vi "getData.vi"(9 "COM":bool, 10 "VISA name":refnum<visa-resource-name>, 11 "Array":string[](array[string])) -> (2 "return":i32, 3 "Numeric":u16)   [LabVIEW 2016]
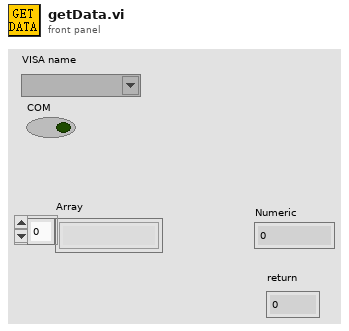
[diagram p1: front panel]
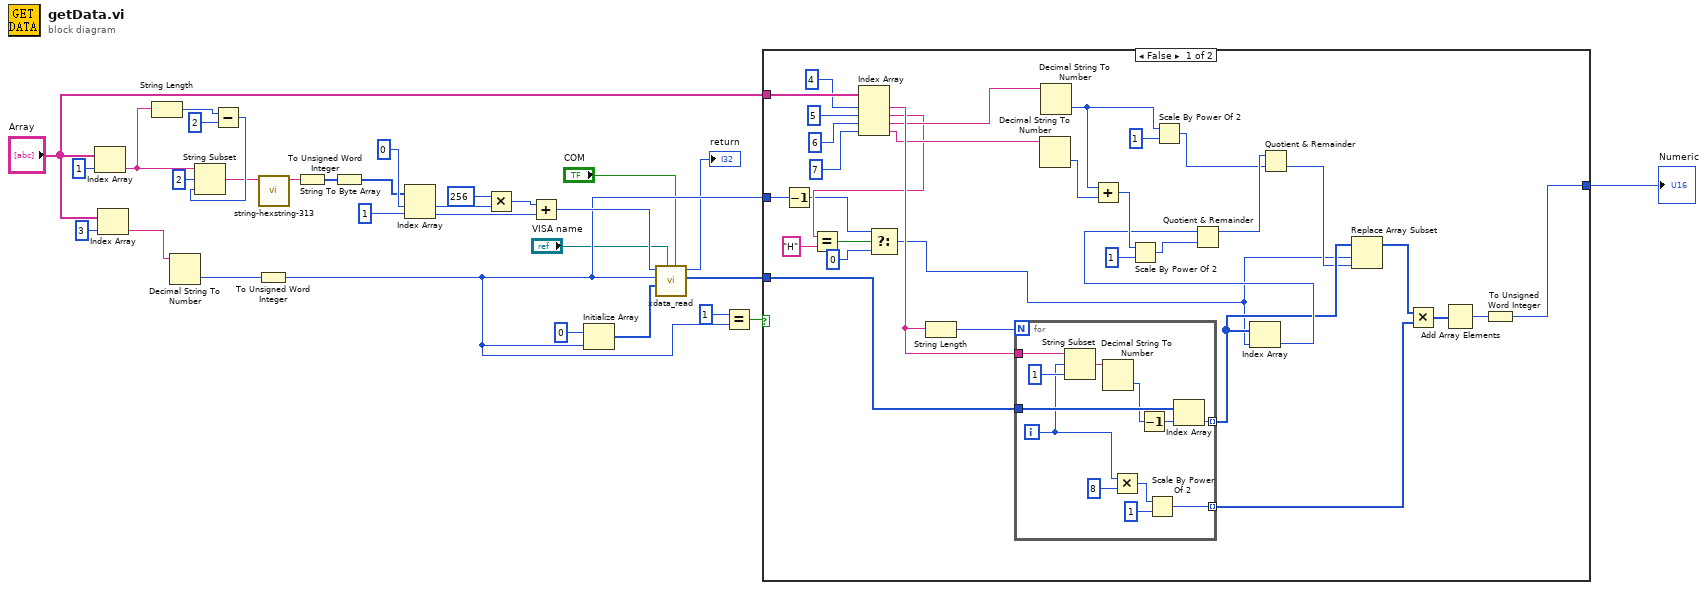
[diagram p0: block diagram]
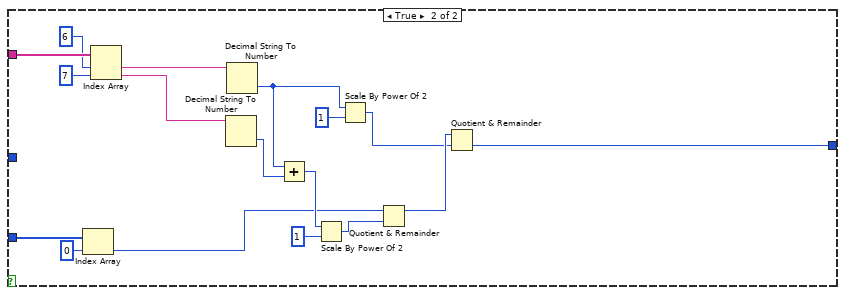
[diagram p2: hidden frame]
diagram:
  n1 = Index Array(array="Array", index=1) -> (element=w30:string)
  n2 = Index Array(array="Array", index=3) -> (element=w14:string)
  n3 = String Length(string=w30) -> (length=w29:i32)
  n4 = Decimal String To Number(string=w14) -> (number=w12:i32)  [unwired: 2 in, 1 out]
  n5 = Subtract(x=w29, y=2) -> (x-y=w27:i32)
  n6 = String Subset(string=w30, offset (0)=2, length (rest)=w27) -> (substring=w25:string)
  n7 = To Unsigned Word Integer(number=w12) -> (unsigned 16bit integer=w4:u16)
  n8 = call "string-hexstring-313.vi"("字符串"=w25) -> ("十六进制整型字符串"=w24:string)  [unwired: 10 in]
  n9 = String To Byte Array(string=w24) -> (unsigned byte array=w23:u8[])
  n10 = To Unsigned Word Integer(number=w23) -> (unsigned 16bit integer=w20:u16[])
  n11 = Index Array(array=w20, index #1=0 ("index"), index #2=1 ("index")) -> (element #1=w19:u16, element #2=w16:u16)
  n12 = Multiply(x=u16 256, y=w19) -> (x*y=w17:u16)
  n13 = Add(x=w17, y=w16) -> (x+y=w13:u16)
  n14 = Initialize Array(u8 0 ("element"), w4) -> (w10:u8[])
  n15 = call "xdata_read.vi"("COM"="COM", "VISA name"="VISA name", "data"=w10, "wLen"=w4, "wAddr"=w13) -> ("data out"=w7:u8[], "return"=→"return":i32)  [unwired: 5 in]
  n16 = Equal?(x=u16 1, y=w4) -> (x = y?=w9:bool)
  n17 = case shown="False" w9 {
    tunnel: w7 -> [w47 w93]
    tunnel: "Array" -> [w64 w91]
    tunnel: [w39 w77] -> w5
    tunnel: w4 -> [w35 _]
    frame False {
      n18 = Decrement(x=w35) -> (x-1=w32:u16)
      n19 = Index Array(array=w64, index #1=4 ("index"), index #2=5 ("index"), index #3=6 ("index"), index #4=7 ("index")) -> (element #1=w50:string, element #2=w38:string, element #3=w49:string, element #4=w48:string)
      n20 = Equal?(x=w38, y="H") -> (x = y?=w36:bool)
      n21 = Select(t=w32, s=w36, f=u16 0) -> (s? t:f=w33:u16)
      n22 = String Length(string=w50) -> (length=w51:i32)
      n23 = for {
        N: w51 -> [_]
        tunnel: w50 -> [w76]
        tunnel: [w71] -> w45 mode=indexing
        tunnel: w47 -> [w73]
        tunnel: [w66] -> w42 mode=indexing
        i -> [w67]
        n24 = String Subset(string=w76, offset (0)=w67, length (rest)=1 ("length (rest)")) -> (substring=w74:string)
        n25 = Decimal String To Number(string=w74) -> (number=w72:i32)  [unwired: 2 in, 1 out]
        n26 = Multiply(x=w67, y=8) -> (x*y=w68:i32)
        n27 = Decrement(x=w72) -> (x-1=w65:i32)
        n28 = Scale By Power Of 2(n=w68, x=1 ("x*y")) -> (x*2^n=w66:i32)
        n29 = Index Array(array=w73, index=w65) -> (element=w71:u8)
      }
      n30 = Decimal String To Number(string=w48) -> (number=w58:i32)  [unwired: 2 in, 1 out]
      n31 = Decimal String To Number(string=w49) -> (number=w59:i32)  [unwired: 2 in, 1 out]
      n32 = Add(x=w59, y=w58) -> (x+y=w57:i32)
      n33 = Scale By Power Of 2(n=w57, x=u16 1) -> (x*2^n=w56:u16)
      n34 = Scale By Power Of 2(n=w59, x=u8 1) -> (x*2^n=w54:u8)
      n35 = Index Array(array=w45, index=w33) -> (element=w46:u8)
      n36 = Quotient & Remainder(x=w46, y=w56) -> (x-y*floor(x/y)=w55:u16)  [unwired: 1 out]
      n37 = Quotient & Remainder(x=w55, y=w54) -> (floor(x/y)=w44:u16)  [unwired: 1 out]
      n38 = Replace Array Subset(array=w45, new element=w44, index=w33) -> (w43:u8[])
      n39 = Multiply(x=w43, y=w42) -> (x*y=w41:i32[])
      n40 = Add Array Elements(numeric array=w41) -> (sum=w40:i32)
      n41 = To Unsigned Word Integer(number=w40) -> (unsigned 16bit integer=w39:u16)
    }
    frame True {
      n42 = Index Array(array=w93, index=0) -> (element=w81:u8)
      n43 = Index Array(array=w91, index #1=6 ("index"), index #2=7 ("index")) -> (element #1=w87:string, element #2=w88:string)
      n44 = Decimal String To Number(string=w88) -> (number=w83:i32)  [unwired: 2 in, 1 out]
      n45 = Decimal String To Number(string=w87) -> (number=w84:i32)  [unwired: 2 in, 1 out]
      n46 = Add(x=w84, y=w83) -> (x+y=w82:i32)
      n47 = Scale By Power Of 2(n=w82, x=u16 1) -> (x*2^n=w80:u16)
      n48 = Scale By Power Of 2(n=w84, x=u8 1) -> (x*2^n=w78:u8)
      n49 = Quotient & Remainder(x=w81, y=w80) -> (x-y*floor(x/y)=w79:u16)  [unwired: 1 out]
      n50 = Quotient & Remainder(x=w79, y=w78) -> (floor(x/y)=w77:u16)  [unwired: 1 out]
    }
  }
  "Numeric" <- w5
